vi "_Add Sheet.vi"(8 "error in":errorcluster, 10 "SheetName":string, 11 "SpreadsheetDoc in":refnum<k24>) -> (0 "error out":errorcluster, 1 "Sheet Index":i32, 2 "Sheet":refnum<k24>, 3 "SpreadsheetDoc out":refnum<k24>)   [LabVIEW 2019, in "Open Xml.lvlib"]
uses:
  Open Xml.lvlib
  D:/git/Open-Xml-LabVIEW/Source/DocumentFormat.OpenXml.dll
  DocumentFormat.OpenXml.dll
  D:/git/Open-Xml-LabVIEW/Source/DocumentFormat.OpenXml.Framework.dll
  DocumentFormat.OpenXml.Framework.dll
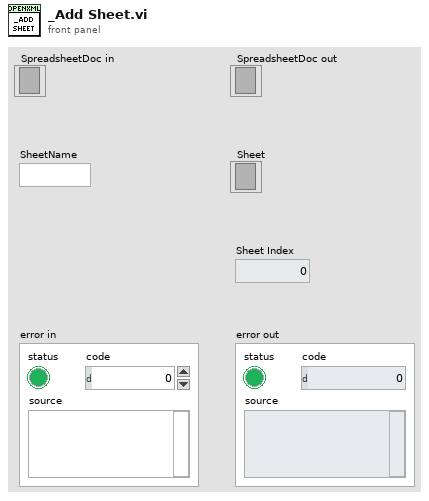
[diagram p1: front panel]
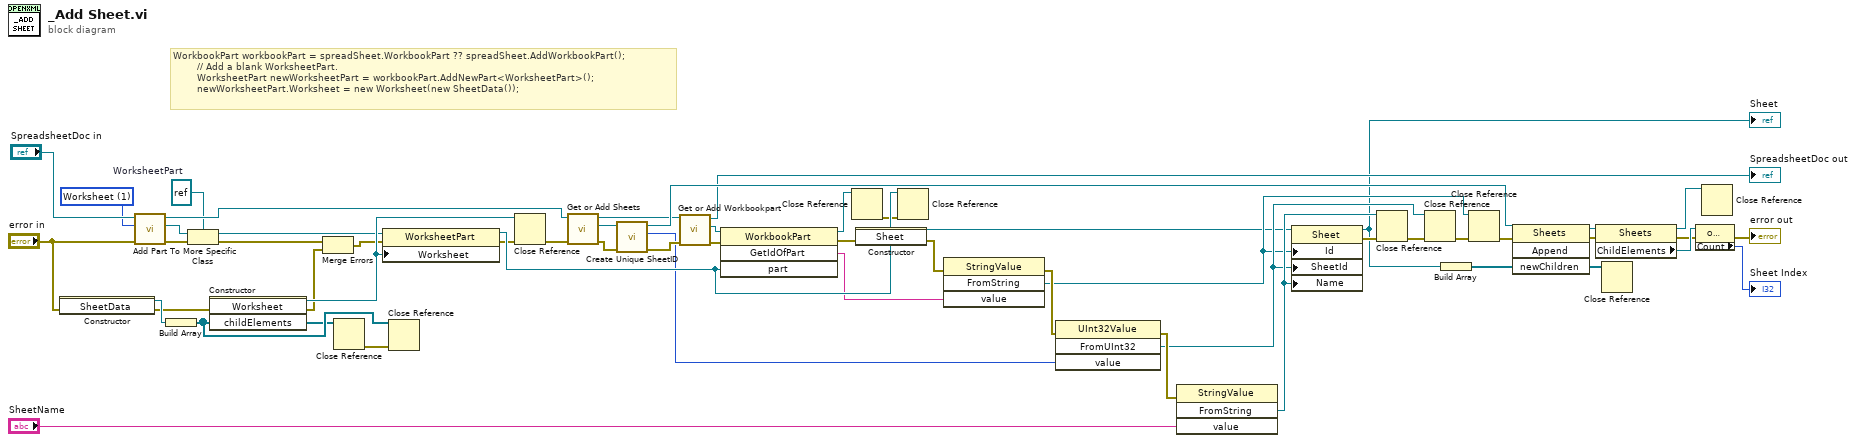
[diagram p0: block diagram]
diagram:
  w11 = 1 items=["SharedString", "Worksheet", "WorkbookStyles"] ("PartType")
  w17 = refnum<k24> refnum  # WorksheetPart
  # "WorkbookPart workbookPart = spreadSheet.WorkbookPart ?? spreadSheet.AddWorkbookPart();\n        // Add a blank WorksheetPart.\n        WorksheetPart newWorksheetPart = workbookPart.AddNewPart<WorksheetPart>();\n        newWorksheetPart.Worksheet = new Worksheet(new SheetData());"
  n1 = constructor class="SheetData"(error in="error in") -> (reference out=w16:refnum<k24>, error out=w15:errorcluster)  [unwired: 2 in, 1 out]
  n2 = call "Add Part.vi"("error in"="error in", "PartType"=w11, "SpreadsheetDoc in"="SpreadsheetDoc in") -> ("error out"=w22:errorcluster, "OpenXmlPart"=w14:refnum<k24>, "SpreadsheetDoc out"=w30:refnum<k24>)  [unwired: 6 in]
  n3 = Build Array(w16) -> (w21:refnum<k24>[])
  n4 = To More Specific Class(target class=w17, reference=w14, error in=w22) -> (specific class reference=w18:refnum<k24>, error out=w23:errorcluster)
  n5 = constructor class="Worksheet"(error in=w15, "childElements"=w21) -> (reference out=w28:refnum<k24>, error out=w26:errorcluster, "childElements"=w20:refnum<k24>[])  [unwired: 2 in, 1 out]
  n6 = Merge Errors(w23, w26) -> (w25:errorcluster)
  n7 = Close Reference(reference=w20) -> (error out=w19:errorcluster)  [unwired: 1 in]
  n8 = property on="New WorksheetPart" class="WorksheetPart"(reference=w18, error in=w25, "Worksheet"=w28) -> (reference out=w50:refnum<k24>, error out=w27:errorcluster)
  n9 = Close Reference(reference=w21, error in (no error)=w19) -> ()  [unwired: 1 out]
  n10 = Close Reference(reference=w28, error in (no error)=w27) -> (error out=w29:errorcluster)
  n11 = call "Get or Add Sheets.vi"("error in"=w29, "SpreadsheetDoc in"=w30) -> ("error out"=w53:errorcluster, "Sheets"=w51:refnum<k24>, "SpreadsheetDoc out"=w33:refnum<k24>)  [unwired: 7 in]
  n12 = call "Create Unique SheetID.vi"("error in"=w53, "Sheets in"=w51) -> ("error out"=w54:errorcluster, "Unique SheetID"=w36:u32, "Sheets out"=w52:refnum<k24>)  [unwired: 7 in]
  n13 = call "Get or Add Workbookpart.vi"("error in"=w54, "SpreadsheetDoc in"=w33) -> ("error out"=w32:errorcluster, "WorkbookPart"=w31:refnum<k24>, "SpreadsheetDoc out"=→"SpreadsheetDoc out":refnum<k24>)  [unwired: 7 in]
  n14 = invoke class="WorkbookPart" method="GetIdOfPart"(reference=w31, error in=w32, "part"=w50) -> (reference out=w55:refnum<k24>, error out=w8:errorcluster, "GetIdOfPart"=w35:string)  [unwired: 1 in, 1 out]
  n15 = Close Reference(reference=w55) -> (error out=w7:errorcluster)  [unwired: 1 in]
  n16 = constructor class="Sheet"(error in=w8) -> (reference out=w34:refnum<k24>, error out=w42:errorcluster)  [unwired: 2 in, 1 out]
  n17 = Close Reference(reference=w50, error in (no error)=w7) -> ()  [unwired: 1 out]
  n18 = invoke class="StringValue" method="FromString"(error in=w42, "value"=w35) -> (error out=w41:errorcluster, "FromString"=w38:refnum<k24>)  [unwired: 2 in, 2 out]
  n19 = invoke class="UInt32Value" method="FromUInt32"(error in=w41, "value"=w36) -> (error out=w43:errorcluster, "FromUInt32"=w40:refnum<k24>)  [unwired: 2 in, 2 out]
  n20 = invoke class="StringValue" method="FromString"(error in=w43, "value"="SheetName") -> ("FromString"=w46:refnum<k24>)  [unwired: 2 in, 3 out]
  n21 = property class="Sheet"(reference=w34, "Id"=w38, "SheetId"=w40, "Name"=w46) -> (reference out=w9:refnum<k24>, error out=w37:errorcluster)  [unwired: 1 in]
  "Sheet" <- w9
  n22 = Close Reference(reference=w46, error in (no error)=w37) -> (error out=w45:errorcluster)
  n23 = Close Reference(reference=w40, error in (no error)=w45) -> (error out=w39:errorcluster)
  n24 = Build Array(w9) -> (w12:refnum<k24>[])
  n25 = Close Reference(reference=w38, error in (no error)=w39) -> (error out=w47:errorcluster)
  n26 = invoke class="Sheets" method="Append"(reference=w52, error in=w47, "newChildren"=w12) -> (reference out=w6:refnum<k24>, error out=w48:errorcluster, "newChildren"=w13:refnum<k24>[])  [unwired: 1 in, 1 out]
  n27 = property class="Sheets"(reference=w6, error in=w48) -> (reference out=w5:refnum<k24>, error out=w2:errorcluster, "ChildElements"=w4:refnum<k24>)
  n28 = Close Reference(reference=w13) -> ()  [unwired: 1 in, 1 out]
  n29 = property class="OpenXmlElementList"(reference=w4, error in=w2) -> (error out=→"error out":errorcluster, "Count"=→"Sheet Index":i32)  [unwired: 1 out]
  n30 = Close Reference(reference=w5) -> ()  [unwired: 1 in, 1 out]
